vi "Create and Save Control.vi"(8 "error in (no error)":errorcluster, 10 "PNG Path":path, 11 "Save Path":path) -> (0 "error out":errorcluster, 3 "dup Save Path out":path)   [LabVIEW 2020]
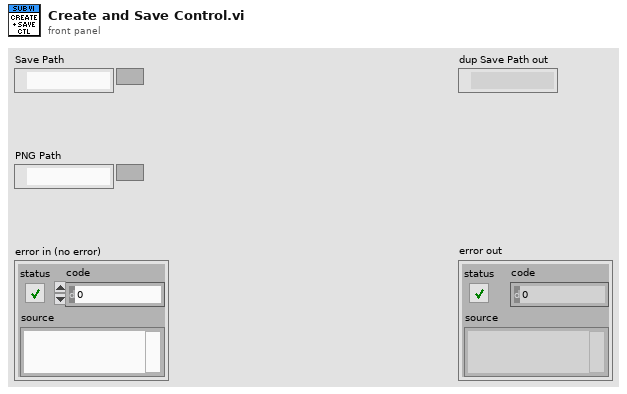
[diagram p1: front panel]
types:
  T1 = cluster{"type":u32, "id":i32, "name":string, "binary data":string}[]
  T2 = cluster{"type":u32, "id":i32, "name":string, "binary data":string}
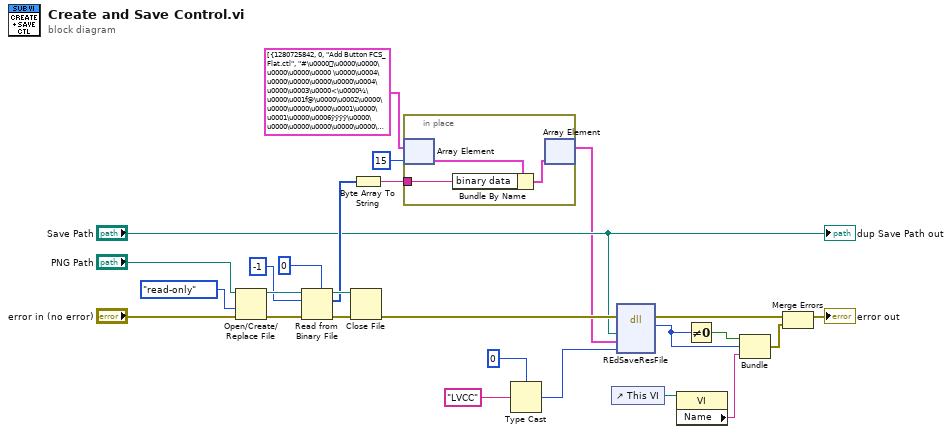
[diagram p0: block diagram]
diagram:
  n1 = Open/Create/Replace File(file path (use dialog)="PNG Path", error in="error in (no error)", access (0:read/write)=enum16{"read/write", "read-only", "write-only"}."read-only") -> (refnum out=w21:refnum<file>, error out=w22:errorcluster)  [unwired: 3 in, 1 out]
  n2 = Read from Binary File(5:u8 0, 8:w22, 10:-1 ("count (1)"), 11:w21) -> (0:w24:errorcluster, 2:w16:u8[], 3:w23:refnum<file>)  [unwired: 2 in, 1 out]
  n3 = Close File(refnum=w23, error in=w24) -> (error out=w14:errorcluster)  [unwired: 1 out]
  n4 = Byte Array To String(unsigned byte array=w16) -> (string=w15:string)
  n5 = in-place {
    in-place-border: w15 -> [w28]
    n6 = in-place-array #1(T1 [{"type"=1280725842, "id"=0, "name"="Add Button FCS_Flat.ctl", "binary data"="#\u0000\u0000\u0000\u0000\u0000\u0000 \u0000\u0004\u0000\u0000\u0000\u0000\u0004\u0000\u0003\u0000<\u0000¼\u0000\u001f@\u0000\u0002\u0000\u0000\u0000\u0000\u0001\u0000\u0001\u0000\u0006ÿÿÿÿ\u0000\u0000\u0000\u0000\u0000\u0000\u0000\u0000\u0000\u0000\u0000\u00000¿c@¿s\u0007óFâ\u0000\u0000\u0000\f\u0000\u0000\u0000\u0010\u0000\u0000\u0000\u0000t)ëãGN\u0002y¦¿ 9Ô\u001dÙ\u0000²\u0004é\tìøB~\u0000\u0000\u0000\u0000\u0000\u0000\u0000\u0000Ù^R5çäEK\u0011mU(\u001aC\u0001\u0000\u0000\u0000ÿÿÿÿÔ\u001dÙ\u0000²\u0004é\tìøB~"}, {"type"=1381258055, "id"=0, "name"="", "binary data"="‚òWÝ¸ðÜ@\u0006O/\u0002P3Š¸"}, {"type"=1279882857, "id"=0, "name"="", "binary data"="\u0000\u0001LVCC\u0000\u0000\u0000\u0000\u0000\u0003"}, {"type"=1129270864, "id"=0, "name"="", "binary data"="\u0000\u0001"}, {"type"=1986359923, "id"=4, "name"="", "binary data"="#6€\u0006\u0000\u0000\u000623.3.6\u0000"}, {"type"=1986359923, "id"=7, "name"="", "binary data"="#\u0000€\u0000\u0000\u0000\u000423.0\u0000"}, {"type"=1986359923, "id"=8, "name"="", "binary data"="#6€\u0006\u0000\u0000\u000623.3.6\u0000"}, {"type"=1986359923, "id"=9, "name"="", "binary data"="#\u0000€\u0000\u0000\u0000\u000423.0\u0000"}, {"type"=1986359923, "id"=10, "name"="", "binary data"="#6€\u0006\u0000\u0000\u000623.3.6\u0000"}, {"type"=1229147982, "id"=0, "name"="", "binary data"="\u0000\u0000\u0000\u0000?ÿÿü@\u0000\u0000\u0002@\u0000\u0000\u0002@\u0000\u0000\u0002@\u0000\u0000\u0002@\u0000\u0000\u0002@\u0000\u0000\u0002@\u0000\u0000\u0002@\u0000\u0000\u0002@\u0000\u0000\u0002@\u0000\u0000\u0002@\u0000\u0000\u0002@\u0000\u0000\u0002@\u0000\u0000\u0002@\u0000\u0000\u0002@\u0000\u0000\u0002@\u0000\u0000\u0002@D>\u0002@\u0000\u0000\u0002@\u0000\u0000\u0002@\u0000\u0000\u0002@\u0002@\u0002@\u0000\u0000\u0002@\u0000\u0000\u0002@\u0000\u0000\u0002@\u0000\u0000\u0002@\u0000\u0000\u0002@\u0000\u0000\u0002@\u0000\u0000\u0002?ÿÿü\u0000\u0000\u0000\u0000"}, {"type"=1768123448, "id"=0, "name"="", "binary data"="\u0000\u0000\u0000\u0000\u0000\u0000\u0000\u0000\u0000\u0000\u0000\u0000\u0000\u0000\u0000\u0000\u0000\u0000\u0000\u0000\u0000\u0000\u0000\u0000\u0000\u0000\u0000\u0000\u0000\u0000\u0000\u0000\u0000öúúúúúúúúúúúúúúúúúúúúúúúúúúúúö\u0000\u0000úøööööööööööööööööööööööööööøú\u0000\u0000úööööööööööööööööööööööööööööú\u0000\u0000úööööööööööööööööööööööööööööú\u0000\u0000úööööööööööööööööööööööööööööú\u0000\u0000úööööööööööööööööööööööööööööú\u0000\u0000úööööööööööööööööööööööööööööú\u0000\u0000úööööööööööööööööööööööööööööú\u0000\u0000úööööööööööö+yyyy+öööööööööööú\u0000\u0000úöööööööööööOy++yOöööööööööööú\u0000\u0000úöööööööööööOUOOUOöööööööööööú\u0000\u0000úöööööööööööOUOOyOöööööööööööú\u0000\u0000úöööööööööööOUOOyOöööööööööööú\u0000\u0000úöööööö+UUUUyUOOyyUUUU+ööööööú\u0000\u0000úööööööUyOOOOOOOOUUUUyUööööööú\u0000\u0000úööööööUUOOOOOUUUUUUUyUööööööú\u0000\u0000úööööööUUOUUUUyyUyyyyyUööööööú\u0000\u0000úööööööUyyyyyyyyyyyyyU..."}, {"type"=1414091852, "id"=0, "name"="", "binary data"="\u0011Add Button (Flat)"}, {"type"=1129333554, "id"=0, "name"="", "binary data"="\u0000\u0001"}, {"type"=1279878768, "id"=0, "name"="", "binary data"="\u0000\u0001FPHP\u0000\u0000\u0000\u0000\u0000\u0003"}, {"type"=1179665784, "id"=0, "name"="", "binary data"="\u0000\u0000\u0000\u0000"}, {"type"=1296975689, "id"=2, "name"="", "binary data"="PNG\r\n\u001a\n\u0000\u0000\u0000\rIHDR\u0000\u0000\u0000\u0018\u0000\u0000\u0000\u0018\b\u0006\u0000\u0000\u0000àw=ø\u0000\u0000\u0000\u0006bKGD\u0000\u0000\u0000\u0000\u0000\u0000ùC»\u0000\u0000\u0000\tpHYs\u0000\u0000\u0000H\u0000\u0000\u0000H\u0000FÉk>\u0000\u0000\u0000\tvpAg\u0000\u0000\u0000\u0018\u0000\u0000\u0000\u0018\u0000xL¥¦\u0000\u0000\u0002aIDATHÇí=h\u0014Q\u0010Ç³·w{9C.¤2\"J\u0010\u0005+A\"\bÂÎÖJ\b(j/¨`\u0017\u000b« \u0011DÔF#J\u0010\u0004B\u001asIÖûØÝ\u0019Ý\u000bÄd4BþðàÍyó÷`Kÿ_}¼êìì­'©îºi>ïí»ðàzÁË\n@µ\u001eØ«÷_.\u0001o6\u0005\u0010\u0004ÚÙw¨{ ÷À\u000e@xñvGÏÇonZ\u0007`Ï¹aCÅ\u0005È{.f¦\u0002è9ÿ\u0010|¿\tÂ\fÌbkï¹ûdWÄÝ>µ>ààà½¿l¯þEÃ\u0000i&×`»\u0002(@\u0010\u0019~\u00181¢#@Óh8\u0019q]Ý§j\u000eÍê\rò9÷Ì\\þ¹\f\u000e\u0002fâªfF\u0000G\u001dÞs¥»«!q>:Û[¨G\u001aìßÝE¹½xÒ\u00003\u0003\u0011¦g*<\u001d\fÒ\u0000Â®\"âyh ÉHàÓ R\"5@PË\u0011E\u0016\u0017!\u000e^>\u000f\u0010¦ydY¬h\u0004\u0011j \u001aC¾/40¶,jª¡\n²T\u000b_ccÿòÝÔì¶B\u000e%y\u0018©×³³³äy­¨ÁB¥ÂøÔ·yÇY<ÂZ-\u0000ðÓ\u0000ÆÆg«õ\u0000\u0001DR1?Pn/\u000ew[3ªðs¡ÊÇÉÁZ=x\u0006\u0000¹\\¶b!\u0015À/\n¾-3\u001a¡V\fL/j\u0006nÆ/o/ÌÆS\u0011Dµ´\nðúÎéæÖI\u0016..."}, {"type"=1179666530, "id"=0, "name"="", "binary data"="\u0000\u0000\u0004¿x­TÍk\u0013A\u0014/Mâ$lè$61Mâ$V0¥x(R<ÔvTKTÚBõà\u0007lÀ´¨­èE/K!z\u0013z\u0017\u0004=äÐ7\t^ö`O\u001eìaiþ\b\u0006\u000b:ov³i±UPÜÃc\u0019~\u001foÞï1\u0000Áw<\u001dèÀs\tÈÛô3'!jÚ\bÐ(3è}¥uàø\u001dp(\u0012Klï\u0006: v\u00195h)ô(A7\u0011ù\u001eAÃ<CbQ\t¦}*~E8\\¼ÍZÈWÃ0ßÀN`IèßØµB`¨\u001a/c\u0007ÐÈ\u0007Váú½åª%Ôi¤Ì2®dD\u00027ìØ#á!E²~ïI¶`¬{@#P¯×\u000fHqTrÛ¸ 8\u000bÄªBë\u000f\u0004q\u001e\u000bçËz\u0016T}\u001fCïlªÞ\u0015éWêIa\u0013hOý\u001b/øV.']Z³Ù$\u001aÕ\u001eí¾!áL±\fÛ3?b7¬m@ÀÆ\u001dÖýÒÝQüxEàb\u0013Cq\u0002ù<ý_2í°\u0017Y\u00184¸\b\u000fÜ\u0010B½\u00100K!àe7¤QãpÂ¤ý¯Ç¦\u000b7Bôiæ¦ÖVWW½@xÑë``¥\u0013ú.öcI\u001c¦\"O\"SQ\u001bTY8\u000fe¸zxäÊS;ê\u0019\u0014f,ã\u0015ö¼¬Ñ\u0001Âô\u0015Ã\u000bçk\u0018Si8\u0001c ûcç®I,\u00103%¤¿Ê\tr\u001d»\u0004~õú\r©Æuo­±3kèÞü\u0004Ar.$¯*/xùþØg\u0005¥}\u0014:mm\u0013ê_CÞþ_Èn·ûÈÞ_U<M«Z¼\tÅ[`ìkîÒ\u0016'\u0002ôR¬ßV\u0012l^\u0018]\"T\u000eeÍv?¬õß\u0014>C2/$$é..."}, {"type"=1179669317, "id"=0, "name"="", "binary data"="\u0000\u0000\u0000\u0017"}, {"type"=1448100944, "id"=0, "name"="", "binary data"="\u0000\u0000\u0000\u0000"}, {"type"=1279877732, "id"=0, "name"="", "binary data"="\u0000\u0001BDHP\u0000\u0000\u0000\u0000\u0000\u0003"}, {"type"=1111770488, "id"=0, "name"="", "binary data"="\u0000\u0000\u0000\u0000"}, {"type"=1111771234, "id"=0, "name"="", "binary data"="\u0000\u0000\u0000rxc``È\u0013`úÇP÷Ià+!ýYÐñ7\u0003\u0003§Àa Í( \t\u0014ýËÀ.¨\r\u0016Ö>¢ËÁ\u0000\u0005ªl\u001c\u001c\u00059À2\u001c-\u001a\fÿÿÿçøzä\u001a\\Å\u0011\u001f8Se<\u0004\u0000\u0014b\u0019\u0000"}, {"type"=1111774021, "id"=0, "name"="", "binary data"="\u0000\u0000\u0000\u0007"}, {"type"=1447646291, "id"=0, "name"="", "binary data"="\u0000\u0000\u0000\u0002\u0000\u0000\u0000\rNI_IconEditor\u0000\u0000\ry#\u0000\u0000\u0000\u0000\u0000\u0001\u0000\u000e@0ÿÿÿÿ\u0004Data\u0000\u0000\u0001\u0000\u0000\u0000\u0000\rW23368006\r\u0000\u0000\u0000\u0000\u0001\u0017\u0015Load & Unload.lvclass\u0000\u0000\u0001\u0000\u0000\u0000\u0000\u0000\t\u0000\u0000\r%\u0001d\u0001dPTH0\u0000\u0000\u0000\u0004\u0000\u0000\u0000\u0000\u0000\u0000\u0000\u0000\u0000\u0000\u0000\u0001\u0000\u0000\u0000\u0001\u000f\rLayer.lvclass\u0000\u0000\u0001\u0000\u0000\u0000\u0000\u0000\u0007\u0000\u0000\f¹\u0000\u0000\u0000\u0000\u0000\u0000\u0000\u0000\u0000\u0000\f\u0000(\u0000\u0000\f\u0000\u0000\f\u0000\u0000\u0000\u0000\u0000\u0000 \u0000 \u0000\u0018\u0000\u0000\u0000\u0000\u0000ÿÿÿ\u0000\u0000ÿÿÿÿÿÿÿÿÿÿÿÿÿÿÿÿÿÿÿÿÿÿÿÿÿÿÿÿÿÿÿÿÿÿÿÿÿÿÿÿÿÿÿÿÿÿÿÿÿÿÿÿÿÿÿÿÿÿÿÿÿÿÿÿÿÿÿÿÿÿÿÿÿÿÿÿÿÿÿÿÿÿÿÿÿÿÿÿÿÿÿÿÿÿÿÿÿÿÿâââwwwwwwwwwwwwwwwwwwwwwwwwwwwwwwwwwwwwwwwwwwwwwwwwwwwwwwwwwwwwwwwwwwwwwwwwwwwwwwwwwwwwâââÿÿÿÿÿÿwwwªªªââââââââââââââââââââââââââââââââââââââââââââââââââââââââââââââââââââââââââââââªªªwwwÿÿÿÿÿÿwwwââââââââââââââââââââââââââââââââââââââââââââââââââââââââââââââââââââââââââââââââââââwwwÿÿÿÿÿÿwwwâââââââ..."}, {"type"=1146374224, "id"=0, "name"="", "binary data"="\u0000\u0002\u0000\b"}, {"type"=1297434948, "id"=0, "name"="", "binary data"="\u0000\u0000\u0001N"}, {"type"=1212765012, "id"=0, "name"="", "binary data"="\u0000\u0000\u0000\u0002\u0000\u0000\u0004\u0000\u0000\u0000\u0000\n\u0000\u0000\u0000\u0000\u0000\u0000\u0000\u0000\u0000\u0000\u0000\u0000\u0000\u0000\u0000\u0000\u0000\u0000\u0000\u0000\u0000\u0000\u0000\u0000\u0000\u0000\u0000\u0000"}, {"type"=1447253072, "id"=0, "name"="", "binary data"="\u0000\u0000\u0000íxeK\u000e@\u0010Dß0 \u001fè\tà\f^\u0000]¸&ÀÅ8nlÄ¥Gö\bqa*étWUW7°¥lêbï\\uèCèî\b\u001480/\u0006;ìÔæMõ·+Yó´Ý)Ä¥óÊi¥'ÌHmï¼\fµ\r\u000f§Ý\\ZÄ`P1:+4æ(CÅÈ\u000fùÂLøg~ÊjÀø¢a­Dt\f\u001dÅBÉF7Ë_\u0011ö"}, {"type"=1179926850, "id"=128, "name"="", "binary data"="\u0000\u0001\u0000\u0002\u0000\u0003\u0000\u0004\u0000\u0000\u0000H\u0000\u000f\u0004\u0000\u0000\u0000\u0000\u000f\u0000Ù\u0000Ô\u0000\u0000\u0000Q\u0000\u000f\u0004\u0000\u0000\u0000\u0000\u000f\u0000Ù\u0000Ô\u0000\u0000\u0000Z\u0000\u000f\u0004\u0000\u0000\u0000\u0000\u000f\u0000Ù\u0000Ô\u0000\u0000\u0000c€\u0000„\u0000€\u0000\u0000\u000f\u0000Ù\u0000Ô\bSegoe UI\bSegoe UI\bSegoe UI\u00010"}] ("Initial Resources 2"), 15) -> (w29:T2)
    n7 = Bundle By Name(cluster=w29, "binary data"=w28) -> (w27:T2)
    n8 = in-place-array #1(w27) -> (w7:T1)  [unwired: 1 out]
  }
  n9 = Type Cast(type=0, x="LVCC" ("File type")) -> (*(type *) &x=w2:i32)
  n10 = control-ref of="This VI"() -> (w3:refnum<vi>)
  n11 = dll-call lib="LabVIEW" fn="REdSaveResFile"(error in=w14, "resource binary file"="Save Path", "resources in"=w7, w2) -> (error out=w10:errorcluster, w5:i32)  [unwired: 5 in, 1 out]
  n12 = property class="VI"(reference=w3) -> ("Name"=w6:string)  [unwired: 1 in, 2 out]
  n13 = Not Equal To 0?(x=w5) -> (x != 0?=w4:bool)
  n14 = Bundle(w4, w5, "Name"=w6) -> (w9:cluster{bool, i32, "Name":string})  [unwired: 1 in]
  n15 = Merge Errors(w10, w9) -> (→"error out":errorcluster)
  "dup Save Path out" <- "Save Path"
